vi "global-TMO for Sync-Rep.vi"() -> ()   [LabVIEW 2017, in "Communicable State Machine.lvlib"]
uses:
  Communicable State Machine.lvlib
panel:
  in  "TMO for Sync-Rep(ms)":i32=5000
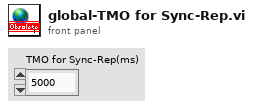
[diagram p1: front panel]
diagram:
